vi "Initialize if Invalid.vi"(8 "error in (no error)":errorcluster, 10 "initialize new if invalid (T)":bool=TRUE, 11 "motor communication in":refnum<class "NI_Robotics_Motor Communication.lvclass">) -> (0 "error out":errorcluster, 2 "initialized new?":bool, 3 "motor communication out":refnum<class "NI_Robotics_Motor Communication.lvclass">)   [LabVIEW 2017, in "NI_Robotics_Motor Communication.lvclass"]
doc: "Initializes a new by-value motor communication object if the input object has not been initialized."
uses:
  <vilib>/robotics/Actuation/Motor Communication/NI_Robotics_Motor Communication.lvclass
  <vilib>/robotics/Actuation/Motor Communication/NI_Robotics_Motor Communication.lvclass/NI_Robotics_Motor Communication.ctl
  <vilib>/robotics/Actuation/Motor Communication Val/NI_Robotics_Motor Communication Val.lvclass
  c:/Program Files (x86)/National Instruments/LabVIEW 2017/vi.lib/robotics/Actuation/Motor Communication/NI_Robotics_Motor Communication.lvclass
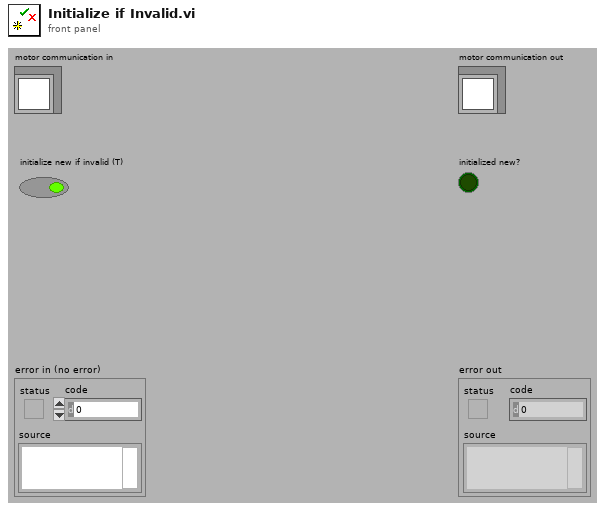
[diagram p1: front panel]
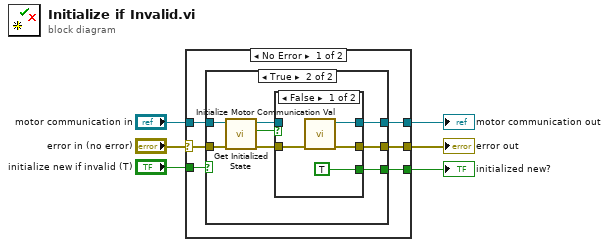
[diagram p0: block diagram]
diagram:
  n1 = case shown="No Error" "error in (no error)" {
    selector: "error in (no error)" -> [w11 w30]
    tunnel: [w9 w30] -> w5
    tunnel: [w10 w29] -> w3
    tunnel: "motor communication in" -> [w12 w29]
    tunnel: [w8 _] -> w2
    tunnel: "initialize new if invalid (T)" -> [w7 _]
    frame No Error {
      n2 = case shown="True" w7 {
        tunnel: w12 -> [w14 w20]
        tunnel: w11 -> [w13 w19]
        tunnel: [w14 w22] -> w10
        tunnel: [w13 w21] -> w9
        tunnel: [_ w15] -> w8
        frame False {
        }
        frame True {
          n3 = call <vilib>:"Get Initialized State.vi"("error in (no error)"=w19, "motor communication in"=w20) -> ("error out"=w16:errorcluster, "initialized"=w18:bool, "motor communication out"=w17:refnum<class "NI_Robotics_Motor Communication.lvclass">)  [unwired: 7 in]
          n4 = case shown="False" w18 {
            tunnel: w17 -> [_ w28]
            tunnel: w16 -> [w26 w27]
            tunnel: [w24 w28] -> w22
            tunnel: [w25 w27] -> w21
            tunnel: [TRUE _] -> w15
            frame False {
              n5 = call <vilib>:"Initialize Motor Communication Val.vi"("error in (no error)"=w26) -> ("error out"=w25:errorcluster, "motor communication val out"=w24:refnum<class "NI_Robotics_Motor Communication Val.lvclass">)  [unwired: 9 in]
            }
            frame True {
            }
          }
        }
      }
    }
    frame Error {
    }
  }
  "error out" <- w5
  "motor communication out" <- w3
  "initialized new?" <- w2
